vi "Part 4 Build Array & Array Subset.vi"() -> ()   [LabVIEW 2020]
panel:
  out "subarray":dbl[](array[numeric])
  in  "array":dbl[](array[numeric])
  out "appended array":dbl[](array[numeric])
  in  "element":dbl
  # "Part 4"
  # "Build Array & Array Subset"
  # "Build Array"
  # "Array Subset"
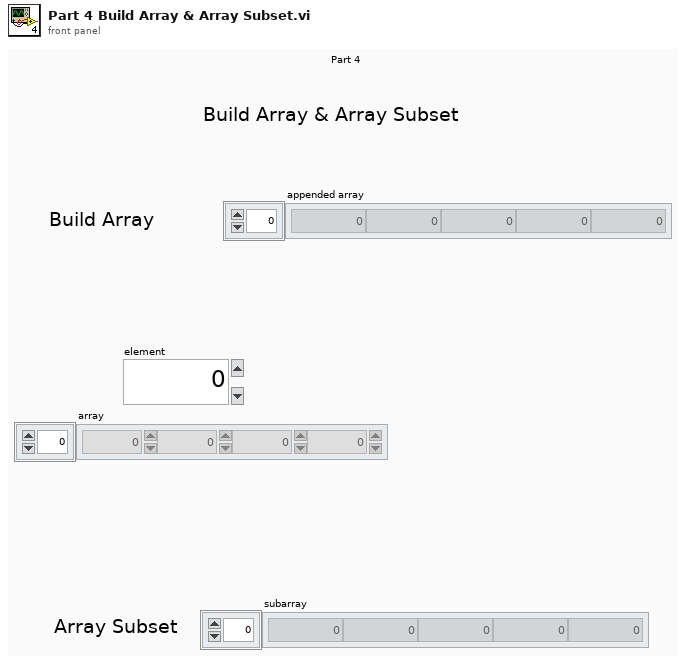
[diagram p1: front panel]
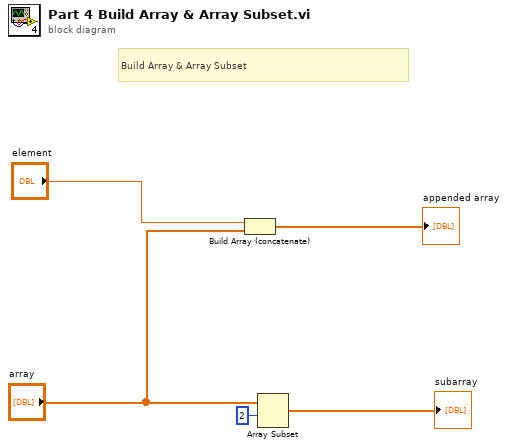
[diagram p0: block diagram]
diagram:
  # "Build Array & Array Subset"
  n1 = Build Array (concatenate) "Build Array"("element", "array") -> (→"appended array":dbl[])
  n2 = Array Subset "Array Subset"(array="array", index=2) -> (→"subarray":dbl[])  [unwired: 1 in]
